vi "Array2Fifo.vi"(8 "Input Array":dbl[](array[numeric]), 11 "DataLoggingParam":T1={"Fifo Size"=0, "FileRefnum"=refnum, "FifoRefnum"=refnum, "Fifo Time Out (ms)"=500, "MaxNumFileWrite"=255, "Force Num Array"=0}) -> ()   [LabVIEW 2010, in "kevLib2011.lvlib"]
uses:
  kevLib2011.lvlib
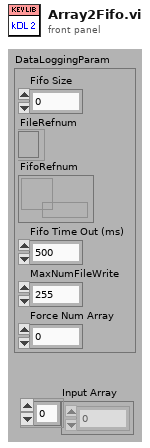
[diagram p1: front panel]
types:
  T1 = cluster{"Fifo Size":u32, "FileRefnum":refnum<file>, "FifoRefnum":refnum<k33>, "Fifo Time Out (ms)":i32, "MaxNumFileWrite":i32, "Force Num Array":i32}
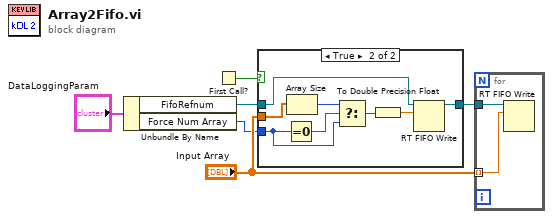
[diagram p0: block diagram]
diagram:
  n1 = Unbundle By Name("DataLoggingParam") -> ("FifoRefnum"=w2:refnum<k33>, "Force Num Array"=w1:i32)
  n2 = First Call?() -> (First Call?: T/F=w6:bool)
  n3 = case shown="True" w6 {
    tunnel: w2 -> [w7 w15]
    tunnel: [w7 w14] -> w4
    tunnel: "Input Array" -> [_ w13]
    tunnel: w1 -> [_ w9]
    frame False {
    }
    frame True {
      n4 = Equal To 0?(x=w9) -> (x = 0?=w11:bool)
      n5 = Array Size(array=w13) -> (size(s)=w10:i32)
      n6 = Select(t=w10, s=w11, f=w9) -> (s? t:f=w8:i32)
      n7 = To Double Precision Float(number=w8) -> (double precision float=w12:dbl)
      n8 = RT FIFO Write(0:w15, 1:w12) -> (8:w14:refnum<k33>)  [unwired: 2 in, 4 out]
    }
  }
  n9 = for {
    tunnel: "Input Array" -> [w16] mode=indexing
    tunnel: w4 -> [w17]
    n10 = RT FIFO Write(0:w17, 1:w16) -> ()  [unwired: 2 in, 5 out]
  }
